vi "zad2.vi"() -> ()   [LabVIEW 2017]
panel:
  in  "Boolean":bool
  in  "stop":bool
  out "Lampa Uliczna":cluster{"1":bool, "2":bool, "3":bool}
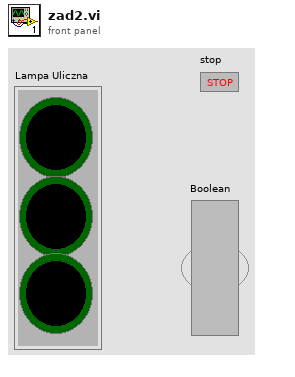
[diagram p1: front panel]
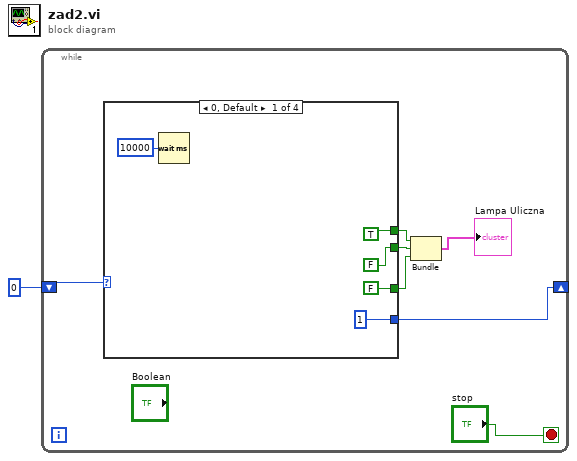
[diagram p0: block diagram]
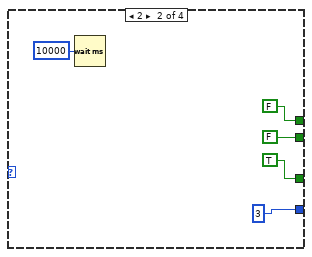
[diagram p2: hidden frame]
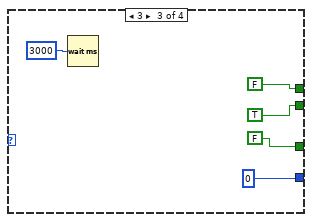
[diagram p3: hidden frame]
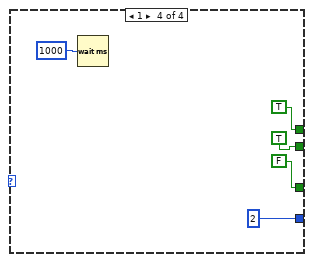
[diagram p4: hidden frame]
diagram:
  n1 = while {
    shift-right: [w2] -> _
    shift-left: 0 -> [w3]
    stop <- "stop" stop-if-true
    n2 = case shown="0, Default" w3 {
      tunnel: [FALSE ("2") FALSE ("2") TRUE ("2") TRUE ("2")] -> w7
      tunnel: [FALSE ("3") TRUE ("3") FALSE ("3") FALSE ("3")] -> w6
      tunnel: [TRUE ("1") FALSE ("1") FALSE ("1") TRUE ("1")] -> w5
      tunnel: [1 3 0 2] -> w2
      frame 0, Default {
        n3 = Wait (ms)(milliseconds to wait=10000) -> ()  [unwired: 1 out]
      }
      frame 2 {
        n4 = Wait (ms)(milliseconds to wait=10000) -> ()  [unwired: 1 out]
      }
      frame 3 {
        n5 = Wait (ms)(milliseconds to wait=3000) -> ()  [unwired: 1 out]
      }
      frame 1 {
        n6 = Wait (ms)(milliseconds to wait=1000) -> ()  [unwired: 1 out]
      }
    }
    n7 = Bundle("1"=w5, "2"=w7, "3"=w6) -> (→"Lampa Uliczna":cluster{"1":bool, "2":bool, "3":bool})  [unwired: 1 in]
  }
